vi "Fdx Close Monitor Queue.vi"(8 "error in":errorcluster, 10 "QueueId":u32, 11 "InstrumentHandle_port in":u32) -> (0 "error out":errorcluster, 3 "InstrumentHandle_port out":u32)   [LabVIEW 2020, in "AIM664LV.lvlib"]
doc: "This function closes the reference to the monitor queue."
uses:
  AIM664LV.lvlib
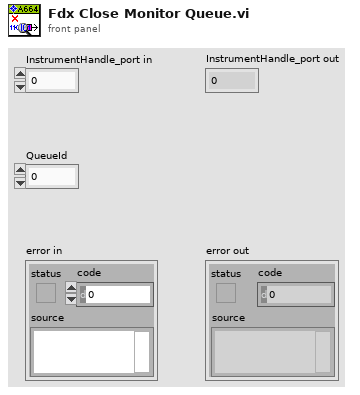
[diagram p1: front panel]
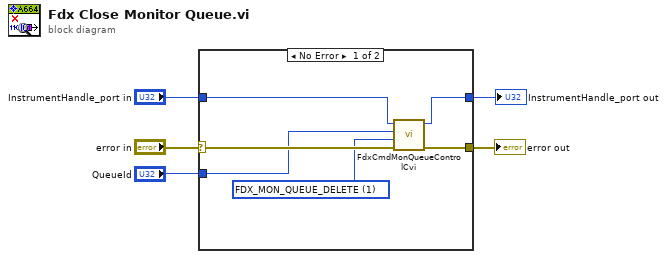
[diagram p0: block diagram]
diagram:
  n1 = case shown="No Error" "error in" {
    selector: "error in" -> [w10 w13]
    tunnel: [w11 w13] -> w4
    tunnel: "QueueId" -> [w7 _]
    tunnel: "InstrumentHandle_port in" -> [w9 w12]
    tunnel: [w8 w12] -> w1
    frame No Error {
      w6 = u32 1 items=["FDX_MON_QUEUE_CREATE", "FDX_MON_QUEUE_DELETE"] ("QueueCtrl")
      n2 = call "FdxCmdMonQueueControlCvi.vi"("error in"=w10, "QueueCtrl"=w6, "QueueId"=w7, "InstrumentHandle_port"=w9) -> ("error out"=w11:errorcluster, "InstrumentHandle_port"=w8:u32)  [unwired: 4 in, 2 out]
    }
    frame Error {
    }
  }
  "error out" <- w4
  "InstrumentHandle_port out" <- w1
